vi "Vision load template.vi"(8 "error in (no error)":errorcluster, 9 "error in":errorcluster, 10 "Step Name":string, 11 "Template Path":path) -> (0 "error out":errorcluster, 2 "error out":errorcluster, 3 "Refnum out":T1)   [LabVIEW 2019]
uses:
  <vilib>/vision/Image Controls.llb/IMAQ Image.ctl
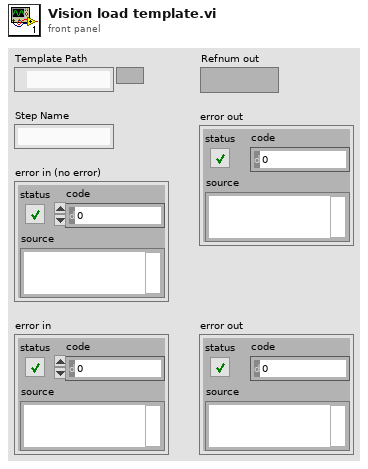
[diagram p1: front panel]
types:
  T1 = typedef "IMAQ Image.ctl" = refnum<image>
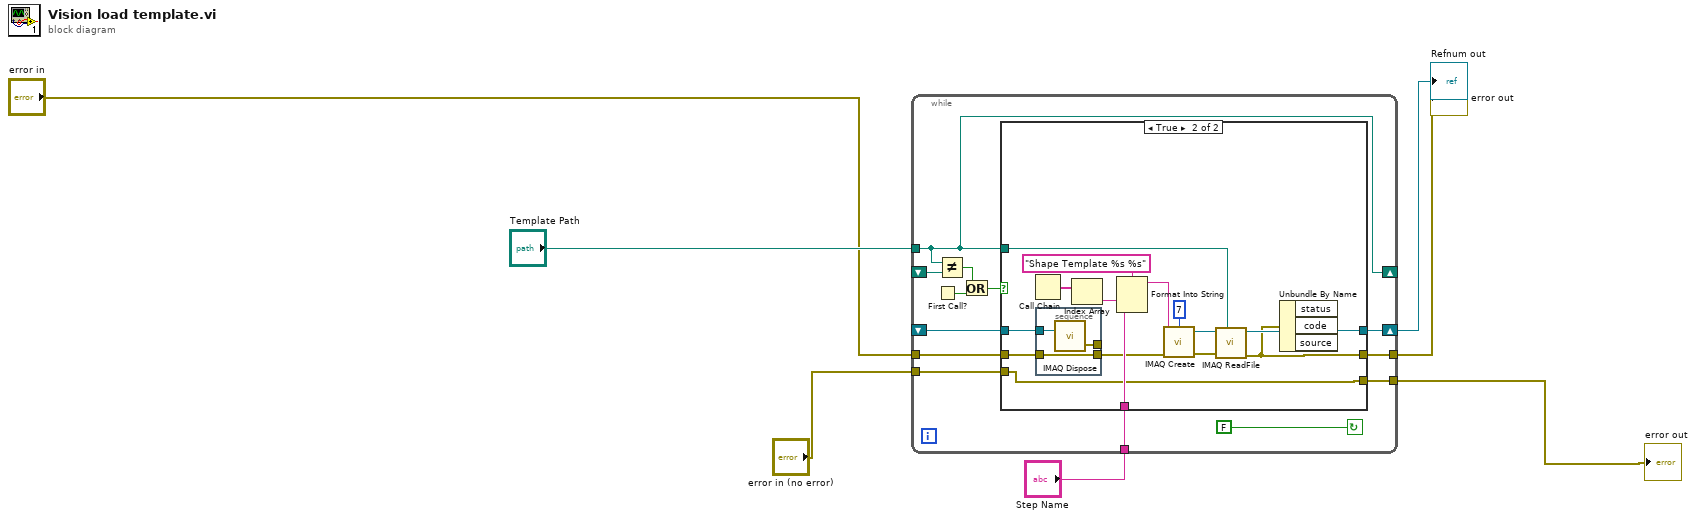
[diagram p0: block diagram]
diagram:
  n1 = while {
    shift-right: [w20] -> w4
    shift-left: _ -> [w19]
    tunnel: [w17] -> w3
    tunnel: "error in" -> [w16]
    tunnel: "Template Path" -> [w14]
    tunnel: "Step Name" -> [w15]
    shift-right: [w14] -> _
    shift-left: _ -> [w13]
    tunnel: [w9] -> w6
    tunnel: "error in (no error)" -> [w8]
    stop <- FALSE continue-if-true
    n2 = First Call?() -> (First Call?: T/F=w12:bool)
    n3 = Not Equal?(x=w14, y=w13) -> (x != y?=w11:bool)
    n4 = Or(x=w11, y=w12) -> (x .or. y?=w10:bool)
    n5 = case shown="True" w10 {
      tunnel: [w23 w35] -> w20
      tunnel: w19 -> [w23 w30]
      tunnel: [w22 w24] -> w17
      tunnel: w16 -> [w22 w29]
      tunnel: w14 -> [_ w25]
      tunnel: w15 -> [_ w31]
      tunnel: [w21 w27] -> w9
      tunnel: w8 -> [w21 w27]
      frame False {
      }
      frame True {
        n6 = Call Chain() -> (call chain=w33:string[])
        n7 = stacked-sequence {
          tunnel: w30 -> [w41]
          tunnel: w29 -> [w40]
          tunnel: [w40] -> w28
          tunnel: [w39] -> _
          frame #0 {
            n8 = call "IMAQ Dispose"("Image"=w41) -> ("error out"=w39:errorcluster)  [unwired: 2 in, 3 out]
          }
        }
        n9 = Index Array(array=w33) -> (element=w32:string)  [unwired: 1 in]
        n10 = Format Into String(format string="Shape Template %s %s" ("Image Name"), w32, w31) -> (resulting string=w38:string)  [unwired: 2 in, 1 out]
        n11 = call "IMAQ Create"("Border Size"=7, "Image Name"=w38, "error in (no error)"=w28) -> ("New Image"=w36:T1, "error out"=w26:errorcluster)  [unwired: 1 in, 1 out]
        n12 = call "IMAQ ReadFile"("File Path"=w25, "error in (no error)"=w26, "Image"=w36) -> ("error out"=w24:errorcluster, "Image Out"=w35:T1)  [unwired: 2 in, 5 out]
        n13 = Unbundle By Name(w24) -> ()  [unwired: 3 out]
      }
    }
  }
  "error out" <- w6
  "Refnum out" <- w4
  "error out" <- w3
